vi "AdafruitSeesawGPIO.vi"() -> ()   [LabVIEW 2020, in "CTI-Scratchpad.lvlib"]
uses:
  CTI-Scratchpad.lvlib
  CTI/Identity.ctl
  CTI/Error Reporting.ctl
  CTI/I2C Address.ctl
  CTI/GPIO Number.ctl
  CTI/I2C Number.ctl
  1a9f6618-71f9-488e-8b4c-ee0cd9edfe5c.vi
  8c02644b-bfa8-40b9-b4d7-1cebf2a2ea64.vi
  CTI/Session/Session.lvclass
  CTI/VisaComms/VisaComms.lvclass
  CTI/CTI.lvlib
  CTI-Peripheral/AdaFruit-Seesaw/AdaFruit-Seesaw.lvclass
panel:
  out "Boolean9":bool
  out "Boolean10":bool
  out "Boolean11":bool
  out "Boolean14":bool
  out "Boolean15":bool
  out "Boolean25":bool
  out "Boolean24":bool
  out "What's Read":bool[](array[boolean])
  out "What's Set":bool[](array[boolean])
  in  "GPIOPin":u16(ring)=9 items=["9"=9, "10"=10, "11"=11, "14"=14, "15"=15, "24"=24, "25"=25]
  in  "Setting":bool
  in  "Stop":bool
  out "loop":i32
  out "Identity":T1
  in  "Grove Connector":enum16{"I2C0", "I2C1"}(ring)
  out "error out":errorcluster
  in  "Port":refnum<visa-resource-name>="COM4"
  # "https://learn.adafruit.com/adafruit-seesaw-atsamd09-breakout/overview"
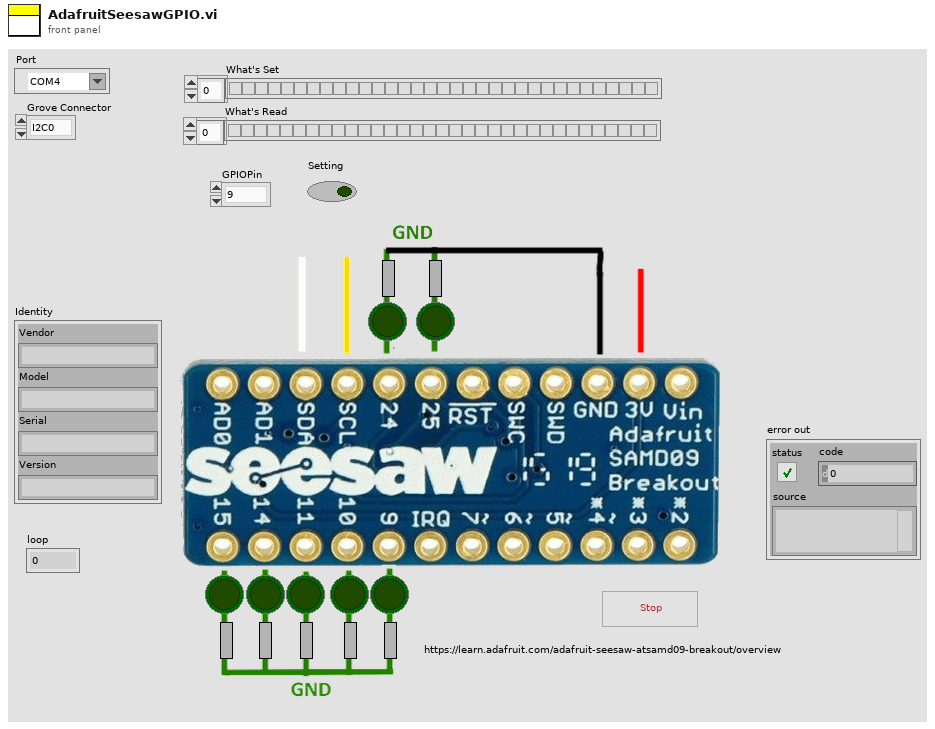
[diagram p1: front panel]
types:
  T1 = typedef "CTI.lvlib/Identity.ctl" = cluster{"Vendor":string, "Model":string, "Serial":string, "Version":string}
  T2 = typedef "CTI.lvlib/I2C Address.ctl" = u8
  T3 = typedef "CTI.lvlib/Error Reporting.ctl" = enum16{"Minimal", "Moderate", "Full"}
  T4 = typedef "CTI.lvlib/I2C Number.ctl" = i8
  T5 = typedef "CTI.lvlib/GPIO Number.ctl" = i8
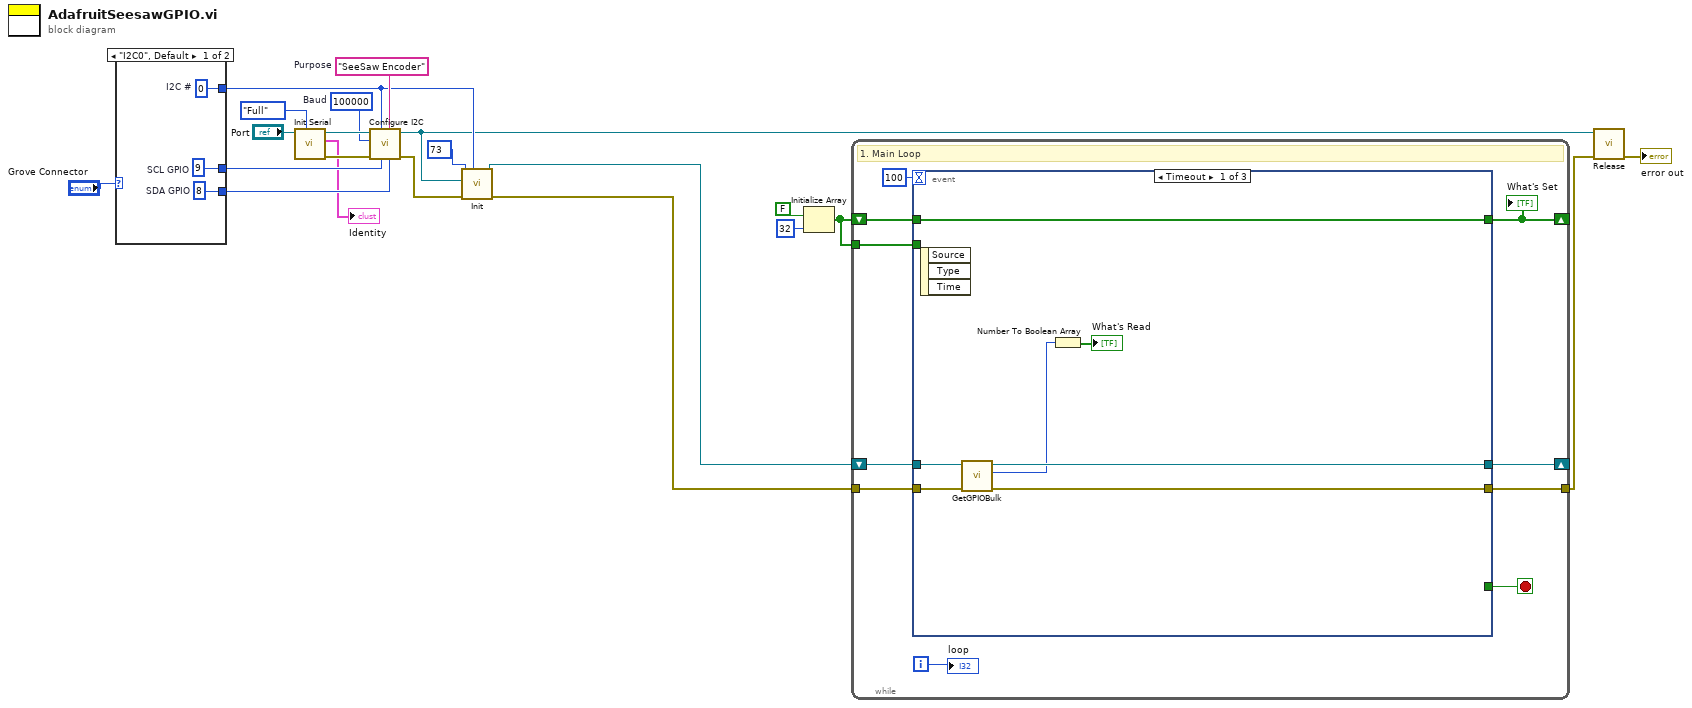
[diagram p0: block diagram]
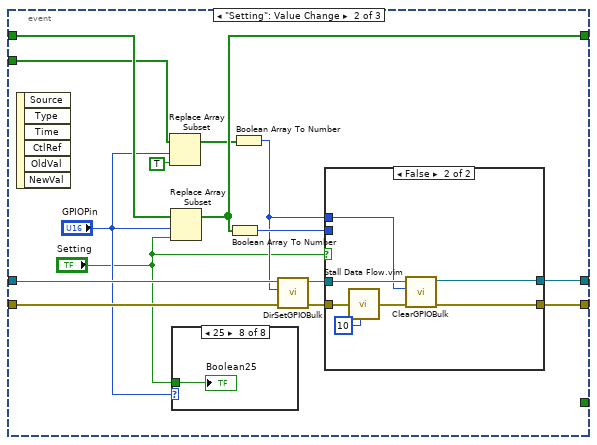
[diagram p2: hidden frame]
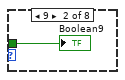
[diagram p4: hidden frame]
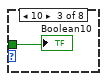
[diagram p5: hidden frame]
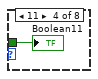
[diagram p6: hidden frame]
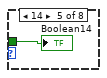
[diagram p7: hidden frame]
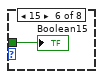
[diagram p8: hidden frame]
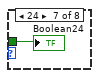
[diagram p9: hidden frame]
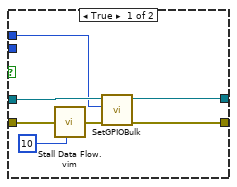
[diagram p10: hidden frame]
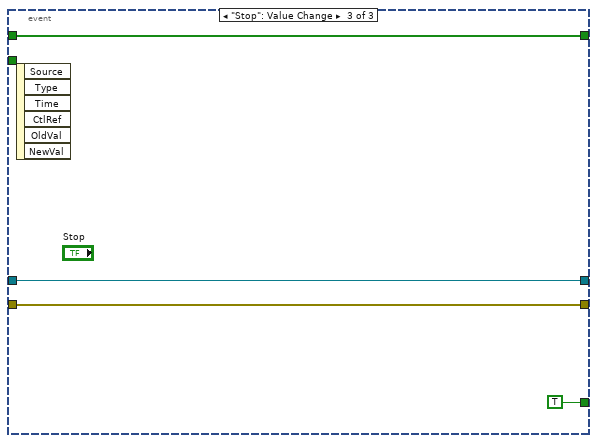
[diagram p11: hidden frame]
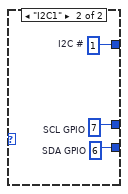
[diagram p12: hidden frame]
diagram:
  w16 = "SeeSaw Encoder"  # Purpose
  w17 = u32 100000  # Baud
  n1 = case shown="\"I2C0\", Default" "Grove Connector" {
    tunnel: [w24 w27] -> w14
    tunnel: [w23 w26] -> w13
    tunnel: [w22 w25] -> w9
    frame "I2C0", Default {
      w22 = T4 0  # I2C #
      w23 = T5 8  # SDA GPIO
      w24 = T5 9  # SCL GPIO
    }
    frame "I2C1" {
      w25 = T4 1  # I2C #
      w26 = T5 6  # SDA GPIO
      w27 = T5 7  # SCL GPIO
    }
  }
  n2 = call "Init Serial.vi"("Error Checking (Full)"=Error_Reporting."Full", "VISA resource name in"="Port") -> ("error out"=w18:errorcluster, "Identity"=→"Identity":T1, "Session"=w19:refnum<class "Session.lvclass">)  [unwired: 7 in]
  n3 = call "Configure I2C.vi"("SDA GPIO"=w13, "Purpose (\"I2C\")"=w16, "SCL GPIO"=w14, "I2C #"=w9, "error in (no error)"=w18, "Baud"=w17, "Session in"=w19) -> ("error out"=w7:errorcluster, "Session out"=w8:refnum<class "Session.lvclass">)  [unwired: 3 in]
  n4 = call "Init.vi"("I2C #"=w9, "error in (no error)"=w7, "Session In"=w8, "Address"=T2 73) -> ("error out"=w5:errorcluster, "AdaFruit-Seesaw out"=w6:refnum<class "AdaFruit-Seesaw.lvclass">)  [unwired: 6 in]
  n5 = Initialize Array(FALSE, 32 ("dimension size")) -> (w1:bool[])
  n6 = while {
    tunnel: w5 -> [w36]
    tunnel: [w34] -> w11
    shift-right: [w31] -> _
    shift-left: w6 -> [w37]
    shift-right: [w29] -> _
    shift-left: w1 -> [w30]
    tunnel: w1 -> [w28]
    i -> [w35]
    stop <- w32 stop-if-true
    # "1. Main Loop"
    n7 = event shown="[0] Timeout" {
      selector: _ -> [_ _ _]
      dyn-events: _ -> [_ _ _]
      timeout: 100 -> [_ _ _]
      tunnel: w37 -> [w43 w53 w82]
      tunnel: w36 -> [w44 w52 w83]
      tunnel: [w41 w56 w83] -> w34
      tunnel: [_ _ TRUE] -> w32
      tunnel: [w42 w57 w82] -> w31
      tunnel: w30 -> [w40 w59 w81]
      tunnel: [w40 w58 w81] -> w29
      tunnel: w28 -> [_ w50 _]
      event Timeout {
        n8 = event-data() -> ()  [unwired: 1 in, 3 out]
        n9 = call "GetGPIOBulk.vi"("error in (no error)"=w44, "AdaFruit-Seesaw in"=w43) -> ("error out"=w41:errorcluster, "GPIO"=w38:u32, "AdaFruit-Seesaw out"=w42:refnum<class "AdaFruit-Seesaw.lvclass">)  [unwired: 7 in]
        n10 = Number To Boolean Array(number=w38) -> (Boolean array=→"What's Read":bool[])
      }
      event "Setting": Value Change {
        n11 = event-data() -> ()  [unwired: 1 in, 6 out]
        n12 = Replace Array Subset(array=w50, new element=TRUE, index="GPIOPin") -> (w48:bool[])
        n13 = Replace Array Subset(array=w59, new element="Setting", index="GPIOPin") -> (w58:bool[])
        n14 = case shown="25" "GPIOPin" {
          tunnel: "Setting" -> [_ w60 w61 w62 w63 w64 w65 w66]
          frame 0, Default {
          }
          frame 9 {
            "Boolean9" <- w60
          }
          frame 10 {
            "Boolean10" <- w61
          }
          frame 11 {
            "Boolean11" <- w62
          }
          frame 14 {
            "Boolean14" <- w63
          }
          frame 15 {
            "Boolean15" <- w64
          }
          frame 24 {
            "Boolean24" <- w65
          }
          frame 25 {
            "Boolean25" <- w66
          }
        }
        n15 = Boolean Array To Number(Boolean array=w58) -> (number=w51:u32)
        n16 = Boolean Array To Number(Boolean array=w48) -> (number=w47:u32)
        n17 = call "DirSetGPIOBulk.vi"("error in (no error)"=w52, "GPIO"=w47, "AdaFruit-Seesaw in"=w53) -> ("error out"=w54:errorcluster, "AdaFruit-Seesaw out"=w55:refnum<class "AdaFruit-Seesaw.lvclass">)  [unwired: 7 in]
        n18 = case shown="False" "Setting" {
          tunnel: [w73 w76] -> w57
          tunnel: [w72 w75] -> w56
          tunnel: w55 -> [w68 w80]
          tunnel: w54 -> [w69 w79]
          tunnel: w51 -> [_ _]
          tunnel: w47 -> [w67 w74]
          frame True {
            n19 = call "Stall Data Flow.vim"("value in"=w69, "milliseconds to wait"=u32 10) -> ("value out"=w71:errorcluster)  [unwired: 1 out]
            n20 = call "SetGPIOBulk.vi"("error in (no error)"=w71, "GPIO"=w67, "AdaFruit-Seesaw in"=w68) -> ("error out"=w72:errorcluster, "AdaFruit-Seesaw out"=w73:refnum<class "AdaFruit-Seesaw.lvclass">)  [unwired: 7 in]
          }
          frame False {
            n21 = call "Stall Data Flow.vim"("value in"=w79, "milliseconds to wait"=u32 10) -> ("value out"=w78:errorcluster)  [unwired: 1 out]
            n22 = call "ClearGPIOBulk.vi"("error in (no error)"=w78, "GPIO"=w74, "AdaFruit-Seesaw in"=w80) -> ("error out"=w75:errorcluster, "AdaFruit-Seesaw out"=w76:refnum<class "AdaFruit-Seesaw.lvclass">)  [unwired: 7 in]
          }
        }
      }
      event "Stop": Value Change {
        n23 = event-data() -> ()  [unwired: 1 in, 6 out]
      }
    }
    "What's Set" <- w29
    "loop" <- w35
  }
  n24 = call-dynamic "Release.vi"("error in (no error)"=w11, "Session in"=w8) -> ("error out"=→"error out":errorcluster)  [unwired: 9 in]
